vi "Send Start Stop to Actors.vi"(8 "error in (no error)":errorcluster, 10 "Start/Stop Acquisition":bool, 11 "Actor Queues":T1) -> (0 "error out":errorcluster)   [LabVIEW 2020, in "Supervisor.lvlib" / "Supervisor.lvclass"]
uses:
  Supervisor.lvclass
  Supervisor.lvclass/Supervisor.ctl
  DAQ AI/DAQ AI Messages/Start Acquisition Msg/Start Acquisition Msg.lvclass
  DAQ AI/DAQ AI Messages/Stop Acquisition Msg/Stop Acquisition Msg.lvclass
  <vilib>/ActorFramework/Message Enqueuer/Message Enqueuer.lvclass
  TypeDef/Actor Queues.ctl
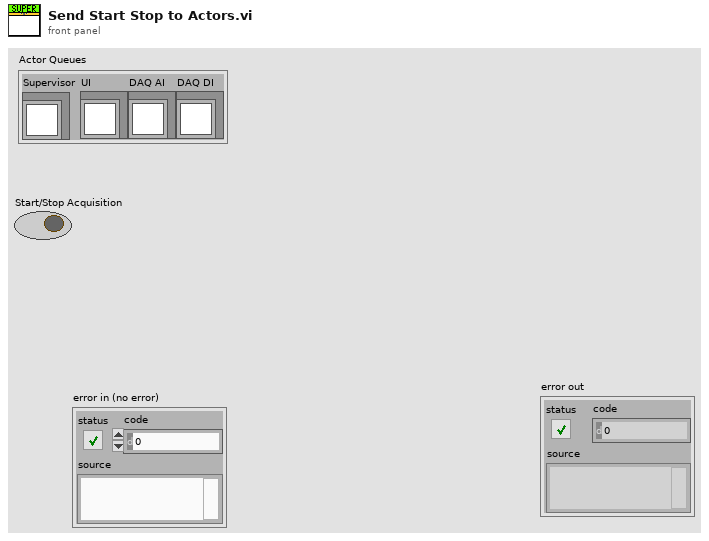
[diagram p1: front panel]
types:
  T1 = typedef "Supervisor.lvlib/Supervisor.lvclass/Actor Queues.ctl" = cluster{"Supervisor":refnum<class "Message Enqueuer.lvclass">, "UI":refnum<class "Message Enqueuer.lvclass">, "DAQ AI":refnum<class "Message Enqueuer.lvclass">, "DAQ DI":refnum<class "Message Enqueuer.lvclass">}
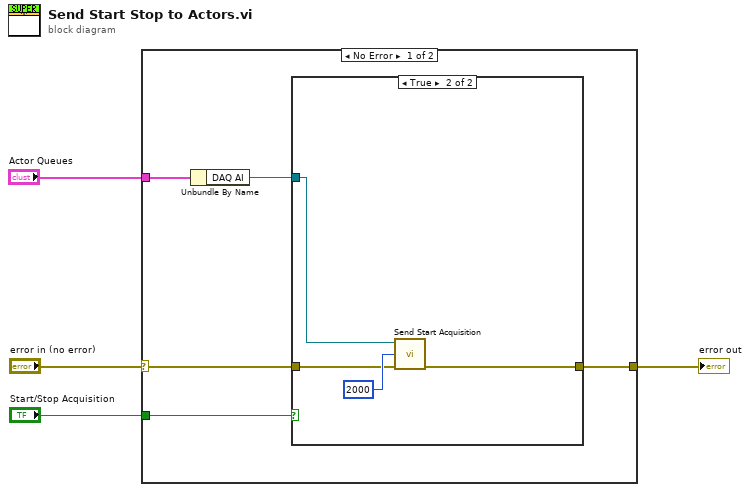
[diagram p0: block diagram]
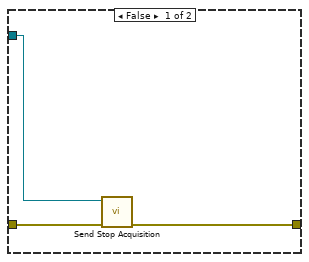
[diagram p2: hidden frame]
diagram:
  n1 = case shown="No Error" "error in (no error)" {
    selector: "error in (no error)" -> [w6 w17]
    tunnel: "Actor Queues" -> [w9 _]
    tunnel: [w5 w17] -> w2
    tunnel: "Start/Stop Acquisition" -> [w8 _]
    frame No Error {
      n2 = Unbundle By Name(w9) -> ("DAQ AI"=w7:refnum<class "Message Enqueuer.lvclass">)
      n3 = case shown="True" w8 {
        tunnel: w7 -> [w11 w16]
        tunnel: w6 -> [w12 w14]
        tunnel: [w10 w13] -> w5
        frame False {
          n4 = call "Send Stop Acquisition.vi"("error in (no error)"=w12, "Message Enqueuer"=w11) -> ("error out"=w10:errorcluster)  [unwired: 8 in, 1 out]
        }
        frame True {
          n5 = call "Send Start Acquisition.vi"("error in (no error)"=w14, "Period [ms]"=2000, "Message Enqueuer"=w16) -> ("error out"=w13:errorcluster)  [unwired: 7 in, 1 out]
        }
      }
    }
    frame Error {
    }
  }
  "error out" <- w2
